vi "VI Tree.vi"   [LabVIEW 2015, in "Siglent SPD3000 Series.lvlib"]
doc: "This is the instrument driver for the Siglent SPD3000 Series Programmable DC Power Supply. The VI Tree displays all the user-callable VIs of the instrument driver in an organized table."
uses:
  <instrlib>/Siglent SPD3000 Series/Siglent SPD3000 Series.lvlib
panel:
  # "(c) 2016 SIGLENT TECHNOLOGIES CO., LTD.   ALL RIGHTS RESERVED."
  # "SEE DIAGRAM\nFOR VI TREE."
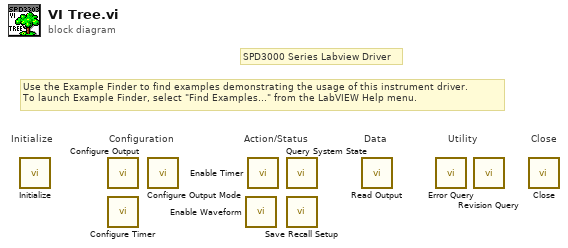
[diagram p0: block diagram]
diagram:
  # "Use the Example Finder to find examples demonstrating the usage of this instrument driver.\nTo launch Example Finder, select \"Find Examples...\" from the LabVIEW Help menu."
  # "SPD3000 Series Labview Driver"
  # "Configuration"
  # "Utility"
  # "Data"
  # "Action/Status"
  # "Close"
  # "Initialize"
  n1 = call <instrlib>:"Initialize.vi"() -> ()  [unwired: 10 in, 2 out]
  n2 = call <instrlib>:"Configure Output.vi"() -> ()  [unwired: 10 in, 2 out]
  n3 = call <instrlib>:"Configure Timer.vi"() -> ()  [unwired: 14 in, 2 out]
  n4 = call <instrlib>:"Configure Output Mode.vi"() -> ()  [unwired: 10 in, 2 out]
  n5 = call <instrlib>:"Enable Waveform.vi"() -> ()  [unwired: 10 in, 2 out]
  n6 = call <instrlib>:"Enable Timer.vi"() -> ()  [unwired: 10 in, 2 out]
  n7 = call <instrlib>:"Query System State.vi"() -> ()  [unwired: 5 in, 7 out]
  n8 = call <instrlib>:"Save Recall Setup.vi"() -> ()  [unwired: 10 in, 2 out]
  n9 = call <instrlib>:"Read Output.vi"() -> ()  [unwired: 8 in, 4 out]
  n10 = call <instrlib>:"Error Query.vi"() -> ()  [unwired: 8 in, 4 out]
  n11 = call <instrlib>:"Revision Query.vi"() -> ()  [unwired: 8 in, 4 out]
  n12 = call <instrlib>:"Close.vi"() -> ()  [unwired: 11 in, 1 out]
